vi "Tbh Inplementation.vi"(0 "Robot Velocities":T3, 1 "Zero V":bool, 2 "Expected Pos":cluster{"x":dbl, "y":dbl, "th":dbl}, 3 "Final Pos":cluster{"x":dbl, "y":dbl, "th":dbl}, 4 "Path Finished?":bool=TRUE) -> (5 "Final velocity":T3, 6 "PID happy":bool=TRUE)   [LabVIEW 2023]
uses:
  swerve/Type Definitions/Data/Robot Velocities.ctl
  Implementation/Tune Alignment PID.ctl
  <vilib>/Rock Robotics/Network Tables/NT Read Numeric Array.vi
panel:
  in  "Disable":cluster{"x":bool, "y":bool, "th":bool}
  in  "Gain":cluster{"x":dbl, "y":dbl, "th":dbl}={"x"=0.25, "y"=0.25, "th"=10.0}
  in  "Invert value":cluster{"x":bool, "y":bool, "th":bool}
  out "Error":cluster{"X":dbl, "Y":dbl, "Theta":dbl}={"X"=0.009854650689625544, "Y"=0.14740072303684304, "Theta"=1.1601458496305803}
  out "Debug Graph":cluster{"sine wave":dbl, "Theta":dbl}(graph)={"sine wave"=-11.72322778883767, "Theta"=-17.14660154582522}
  in  "Debug Input":T2={"amplitude \n(ft or degrees)"=20.0, "frequency (sec)"=0.1, "Tune Align"=enum."Not Enabled"} {"frequency (sec)" format="%0.2f"; "amplitude \n(ft or degrees)" format="%0.2f"}
  in  "Deadband":cluster{"x":dbl, "y":dbl, "th":dbl}={"x"=0.25, "y"=0.25, "th"=10.0}
  # "Half Back Control"
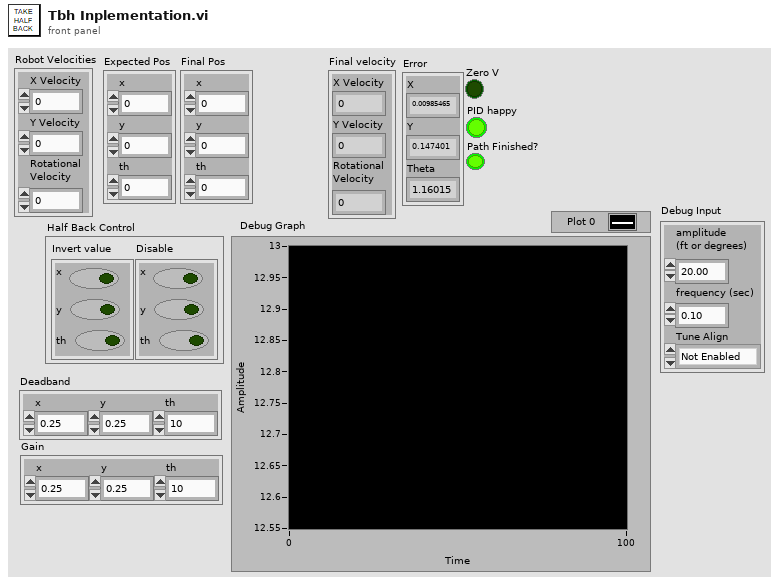
[diagram p1: front panel]
types:
  T1 = typedef "Tune Alignment PID.ctl" = enum16{"Not Enabled", "X Axis", "Y Axis", "Theta"}
  T2 = cluster{"amplitude \n(ft or degrees)":dbl, "frequency (sec)":dbl, "Tune Align":T1}
  T3 = typedef "Robot Velocities.ctl" = cluster{"X Velocity":dbl, "Y Velocity":dbl, "Rotational \nVelocity":dbl}
  T4 = cluster{"Actual":cluster{"x":dbl, "y":dbl, "th":dbl}, "Current":cluster{"x":dbl, "y":dbl, "th":dbl}, "Gain":cluster{"x":dbl, "y":dbl, "th":dbl}}
  T5 = enum16{"X Correction", "Y Correction", "Theta Correction"}
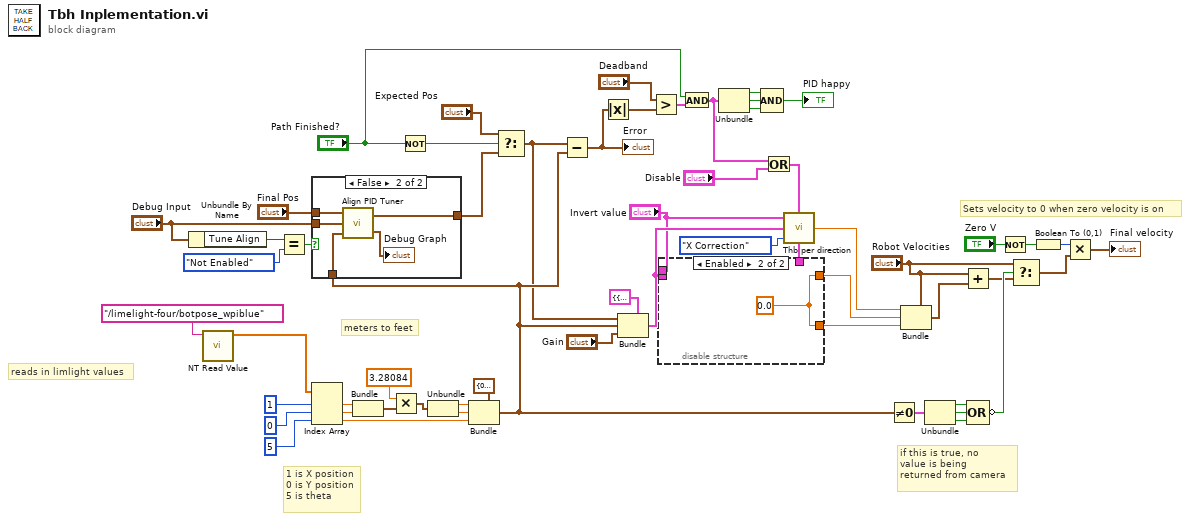
[diagram p0: block diagram]
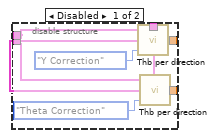
[diagram p2: hidden frame]
diagram:
  # "meters to feet"
  # "reads in limlight values"
  # "1 is X position\n0 is Y position\n5 is theta"
  # "if this is true, no \nvalue is being \nreturned from camera"
  # "Sets velocity to 0 when zero velocity is on"
  n1 = Unbundle By Name("Debug Input") -> ("Tune Align"=w44:T1)
  n2 = call-poly <vilib>:"NT Read Value.vi"("name"="/limelight-four/botpose_wpiblue") -> ("value"=w34:dbl[])  [unwired: 8 in, 2 out]
  n3 = Equal?(x=w44, y=Tune_Alignment_PID."Not Enabled") -> (x = y?=w45:bool)
  n4 = Index Array(array=w34, index #1=1 ("index"), index #2=0 ("index"), index #3=5 ("index")) -> (element #1=w29:dbl, element #2=w28:dbl, element #3=w37:dbl)
  n5 = Bundle("Numeric"=w29, "Numeric"=w28) -> (w33:cluster{"Numeric":dbl, "Numeric":dbl})  [unwired: 1 in]
  n6 = Multiply(x=3.28084, y=w33) -> (x*y=w32:cluster{"Numeric":dbl, "Numeric":dbl})
  n7 = Not(x="Path Finished?") -> (.not. x?=w26:bool)
  n8 = Unbundle(w32) -> ("Numeric"=w31:dbl, "Numeric"=w30:dbl)
  n9 = Bundle(cluster=cluster{"X":dbl, "Y":dbl, "Theta":dbl} {"X"=0.0, "Y"=0.0, "Theta"=0.0}, "X"=w31, "Y"=w30, "Theta"=w37) -> (w11:cluster{"X":dbl, "Y":dbl, "Theta":dbl})
  n10 = case shown="False" w45 {
    tunnel: "Debug Input" -> [_ w60]
    tunnel: "Final Pos" -> [w58 w61]
    tunnel: [w58 w62] -> w41
    tunnel: w11 -> [_ w59]
    frame True {
    }
    frame False {
      n11 = call "Align PID Tuner.vi"("Current Position"=w59, "Debug Input"=w60, "Final Position"=w61) -> ("Graph Data"=→"Debug Graph":cluster{"Error":dbl, "Exppected":dbl}, "Sine Corrected Positions"=w62:cluster{"X":dbl, "Y":dbl, "Theta":dbl})
    }
  }
  n12 = Select(t="Expected Pos", s=w26, f=w41) -> (s? t:f=w10:cluster{"X":dbl, "Y":dbl, "Theta":dbl})
  n13 = Subtract(x=w10, y=w11) -> (x-y=w15:cluster{"X":dbl, "Y":dbl, "Theta":dbl})
  "Error" <- w15
  n14 = Absolute Value(x=w15) -> (abs(x)=w49:cluster{"X":dbl, "Y":dbl, "Theta":dbl})
  n15 = Bundle(cluster=T4 {"Actual"={"x"=0.0, "y"=0.0, "th"=0.0}, "Current"={"x"=0.0, "y"=0.0, "th"=0.0}, "Gain"={"x"=0.0, "y"=0.0, "th"=0.0}} ("Tbh data"), "Actual"=w10, "Current"=w11, "Gain"="Gain") -> (w9:T4)
  n16 = Greater?(x="Deadband", y=w49) -> (0:w24:cluster{bool, bool, bool})
  n17 = And(x="Path Finished?", y=w24) -> (x .and. y?=w1:cluster{bool, bool, bool})
  n18 = Unbundle(w1) -> (w47:bool, w51:bool, w50:bool)
  n19 = Compound Arithmetic op=AND(w47, w51, w50) -> (→"PID happy":bool)
  n20 = Or(x=w1, y="Disable") -> (x .or. y?=w2:cluster{bool, bool, bool})
  n21 = disable-structure shown="Enabled" {
    disable-tunnel: w9 -> [w68 _]
    disable-tunnel: "Invert value" -> [w67 _]
    disable-tunnel: [w66 w71] -> w6
    disable-tunnel: [w65 w71] -> w5
    disable-tunnel: w2 -> [w64 _]
    frame Disabled {
      n22 = call "Thb per direction.vi"("Done?"=w64, "Direction"=T5."Y Correction", "Tbh data"=w68, "Invert value"=w67) -> ("Velocity Ajustment"=w66:dbl)
      n23 = call "Thb per direction.vi"("Done?"=w64, "Direction"=T5."Theta Correction", "Tbh data"=w68, "Invert value"=w67) -> ("Velocity Ajustment"=w65:dbl)
    }
    frame Enabled {
      w71 = 0.0 ("Velocity Ajustment")
    }
  }
  n24 = call "Thb per direction.vi"("Done?"=w2, "Direction"=T5."X Correction", "Tbh data"=w9, "Invert value"="Invert value") -> ("Velocity Ajustment"=w7:dbl)
  n25 = Not Equal To 0?(x=w11) -> (x != 0?=w55:cluster{"X":bool, "Y":bool, "Theta":bool})
  n26 = Bundle(cluster="Robot Velocities", "X Velocity"=w7, "Y Velocity"=w6, "Rotational \nVelocity"=w5) -> (w18:T3)
  n27 = Unbundle(w55) -> ("X"=w54:bool, "Y"=w53:bool, "Theta"=w52:bool)
  n28 = Add(x="Robot Velocities", y=w18) -> (x+y=w19:T3)
  n29 = Compound Arithmetic op=OR(w54, w53, w52) -> (invert w20:bool)
  n30 = Not(x="Zero V") -> (.not. x?=w56:bool)
  n31 = Select(t="Robot Velocities", s=w20, f=w19) -> (s? t:f=w17:T3)
  n32 = Boolean To (0,1)(Boolean=w56) -> (0, 1=w21:i16)
  n33 = Multiply(x=w21, y=w17) -> (x*y=→"Final velocity":T3)
